vi "CreateRoot.vi"(9 "InnerLayers":T1[](array[typedef]), 10 "Alias":string, 11 "Root":refnum<class "Actor.lvclass">) -> ()   [LabVIEW 2020, in "jettl.lvlib"]
uses:
  jettl.lvlib
  CreateRootCore.vi
  Actor/Actor.lvclass
  ActorMap.ctl
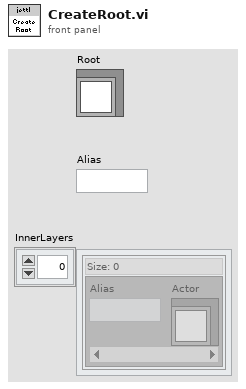
[diagram p1: front panel]
types:
  T1 = typedef "jettl.lvlib/ActorMap.ctl" = map{string, refnum<class "Actor.lvclass">}
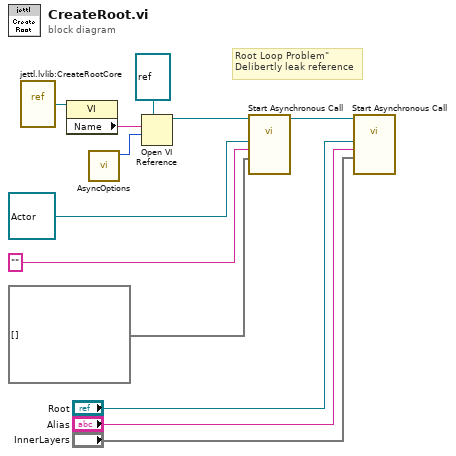
[diagram p0: block diagram]
diagram:
  # "Root Loop Problem\"\nDelibertly leak reference"
  n1 = vi-ref "jettl.lvlib:CreateRootCore.vi"() -> (w11:refnum<vi>)
  n2 = property class="VI"(reference=w11) -> ("Name"=w12:string)  [unwired: 1 in, 2 out]
  n3 = call "AsyncOptions.vi"() -> ("AsyncOptions"=w6:i32)  [unwired: 11 in]
  n4 = Open VI Reference(type specifier VI Refnum (for type only)=refnum<vi> refnum, vi path=w12, options=w6) -> (vi reference=w5:refnum<vi>)  [unwired: 3 in, 1 out]
  n5 = call-by-ref "Start Asynchronous Call"(reference=w5, "Persistent"=T1[] [], "MediatorAlias"="", "Mediator"=refnum<class "Actor.lvclass"> refnum) -> (reference out=w4:refnum<vi>)  [unwired: 10 in, 1 out]
  n6 = call-by-ref "Start Asynchronous Call"(reference=w4, "Persistent"="InnerLayers", "MediatorAlias"="Alias", "Mediator"="Root") -> ()  [unwired: 10 in, 2 out]
